vi "Outward.vi"(11 "64 in":refnum<class "Border.lvclass">) -> (1 "Direction":i32, 2 "Replicated out":refnum<class "Border.lvclass">, 3 "64 out":refnum<class "Border.lvclass">)   [LabVIEW 2015, in "Border.lvclass"]
uses:
  Border.lvclass
  Type Defs/Direction Enum.ctl
  Border.lvclass/Border.ctl
  SubVIs/Read-Only Globals.vi
  SubVIs/Globals (private).vi
  Square/Square.lvclass
  Type Defs/SB Type Defs.lvlib
  Common/Common.lvlib
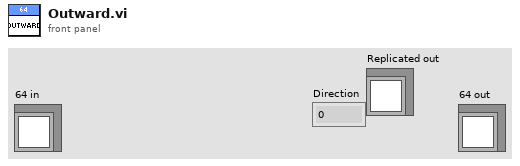
[diagram p1: front panel]
types:
  T1 = typedef "SB Type Defs.lvlib/Direction Enum.ctl" = enum16{"NW", "N", "NE", "E", "SE", "S", "SW", "W"}
  T2 = typedef "Common.lvlib/Position.ctl" = cluster{"Column":i32, "Row":i32}
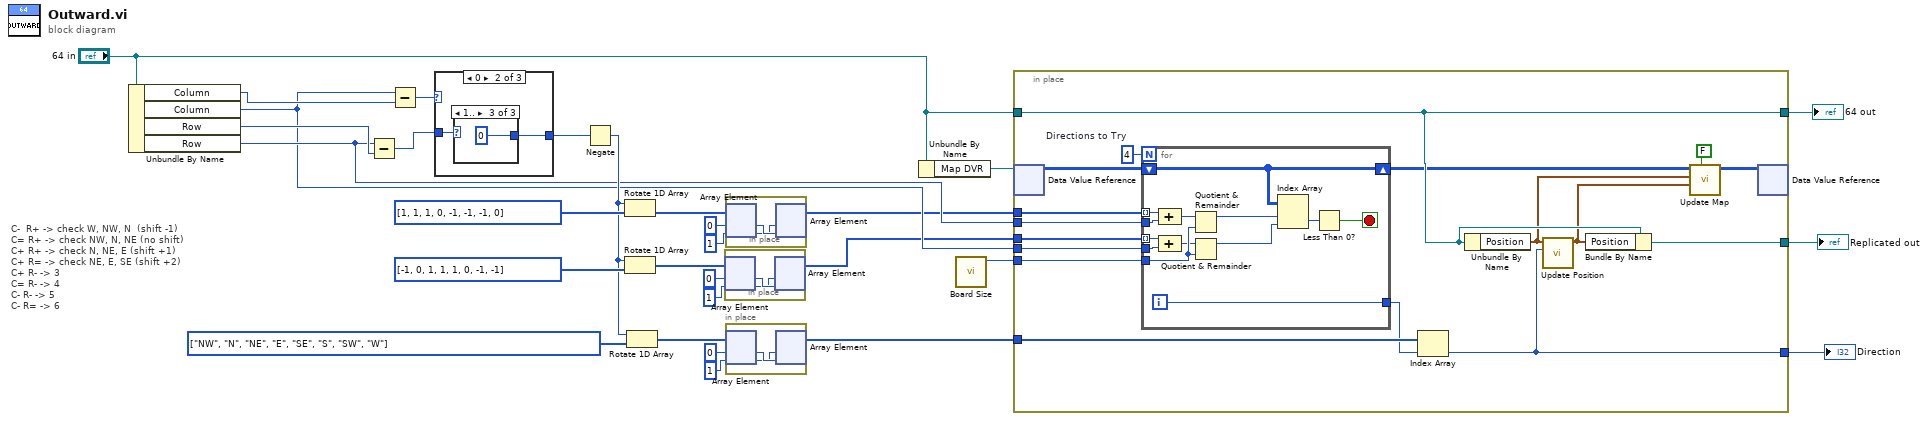
[diagram p0: block diagram]
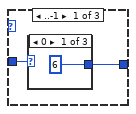
[diagram p2: hidden frame]
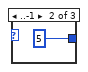
[diagram p3: hidden frame]
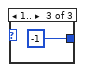
[diagram p4: hidden frame]
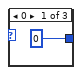
[diagram p5: hidden frame]
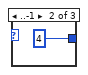
[diagram p6: hidden frame]
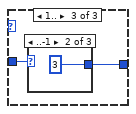
[diagram p7: hidden frame]
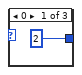
[diagram p8: hidden frame]
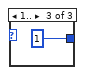
[diagram p9: hidden frame]
diagram:
  w22 = T1[] [enum."NW", enum."N", enum."NE", enum."E", enum."SE", enum."S", enum."SW", enum."W"] items=["NW", "N", "NE", "E", "SE", "S", "SW", "W"]
  # "C-  R+ -> check W, NW, N  (shift -1)\nC= R+ -> check NW, N, NE (no shift)\nC+ R+ -> check N, NE, E (shift +1)\nC+ R= -> check NE, E, SE (shift +2)\nC+ R- -> 3\nC= R- -> 4\nC- R- -> 5\nC- R= -> 6"
  n1 = Unbundle By Name("64 in") -> ("Column"=w29:i32, "Column"=w18:i32, "Row"=w23:i32, "Row"=w19:i32)
  n2 = Subtract(x=w19, y=w23) -> (x-y=w24:i32)
  n3 = Subtract(x=w18, y=w29) -> (x-y=w25:i32)
  n4 = case shown="0" w25 {
    tunnel: w24 -> [w31 w36 w41]
    tunnel: [w30 w35 w40] -> w13
    frame ..-1 {
      n5 = case shown="0" w31 {
        tunnel: [6 5 -1] -> w30
        frame 0 {
        }
        frame ..-1 {
        }
        frame 1.. {
        }
      }
    }
    frame 0 {
      n6 = case shown="1.." w36 {
        tunnel: [0 4 0] -> w35
        frame 0 {
        }
        frame ..-1 {
        }
        frame 1.. {
        }
      }
    }
    frame 1.. {
      n7 = case shown="..-1" w41 {
        tunnel: [2 3 1] -> w40
        frame 0 {
        }
        frame ..-1 {
        }
        frame 1.. {
        }
      }
    }
  }
  n8 = Negate(x=w13) -> (-x=w20:i32)
  n9 = Rotate 1D Array(1:i32[] [1, 1, 1, 0, -1, -1, -1, 0], 2:w20) -> (0:w10:i32[])
  n10 = Rotate 1D Array(1:i32[] [-1, 0, 1, 1, 1, 0, -1, -1], 2:w20) -> (0:w8:i32[])
  n11 = Rotate 1D Array(1:w22, 2:w20) -> (0:w12:T1[])
  n12 = in-place {
    n13 = in-place-array #1(w8, 0, 1) -> (w46:i32, w45:i32)
    n14 = in-place-array #1(w45, w46) -> (w7:i32[])  [unwired: 2 out]
  }
  n15 = in-place {
    n16 = in-place-array #2(w10, 0, 1) -> (w48:i32, w47:i32)
    n17 = in-place-array #2(w47, w48) -> (w9:i32[])  [unwired: 2 out]
  }
  n18 = in-place {
    n19 = in-place-array #3(w12, 0, 1) -> (w50:T1, w49:T1)
    n20 = in-place-array #3(w49, w50) -> (w11:T1[])  [unwired: 2 out]
  }
  n21 = Unbundle By Name("64 in") -> ("Map DVR"=w17:refnum<data-value>)
  n22 = call "Board Size.vi"() -> ("Board Size"=w28:i32)  [unwired: 11 in]
  n23 = in-place {
    in-place-border: w28 -> [w67]
    in-place-border: w9 -> [w66]
    in-place-border: w7 -> [w65]
    in-place-border: w11 -> [w63]
    in-place-border: [w57] -> w21
    in-place-border: w19 -> [w61]
    in-place-border: w18 -> [w60]
    in-place-border: "64 in" -> [w56]
    in-place-border: [w56] -> w15
    in-place-border: [w58] -> w14
    w64 = 4  # Directions to Try
    n24 = in-place-dvr #4(w17) -> (w59:i32[][])  [unwired: 1 out]
    n25 = for {
      N: w64 -> [_]
      tunnel: w66 -> [w80] mode=indexing
      tunnel: w65 -> [w79] mode=indexing
      tunnel: w67 -> [w78]
      tunnel: [w75] -> w62
      tunnel: w61 -> [w71]
      tunnel: w60 -> [w70]
      shift-right: [w68] -> w55
      shift-left: w59 -> [w68]
      i -> [w75]
      stop <- w72 stop-if-true
      n26 = Compound Arithmetic op=ADD(w80, w71) -> (w77:i32)
      n27 = Compound Arithmetic op=ADD(w79, w70) -> (w76:i32)
      n28 = Quotient & Remainder(x=w77, y=w78) -> (x-y*floor(x/y)=w74:i32)  [unwired: 1 out]
      n29 = Quotient & Remainder(x=w76, y=w78) -> (x-y*floor(x/y)=w73:i32)  [unwired: 1 out]
      n30 = Index Array(array=w68, index (row)=w74, index (col)=w73) -> (element=w69:i32)
      n31 = Less Than 0?(x=w69) -> (x < 0?=w72:bool)
    }
    n32 = Index Array(array=w63, index=w62) -> (element=w57:T1)
    n33 = Unbundle By Name(w56) -> ("Position"=w53:T2)
    n34 = call "Update Position.vi"("Direction"=w57, "Position in"=w53) -> ("Position out"=w52:T2)  [unwired: 9 in]
    n35 = Bundle By Name(cluster=w56, "Position"=w52) -> (w58:refnum<class "Border.lvclass">)
    n36 = call "Update Map.vi"("Moved?"=FALSE, "New Position"=w52, "Old Position"=w53, "Map in"=w55) -> ("Map"=w54:i32[][])  [unwired: 7 in]
    n37 = in-place-dvr #4(w54) -> ()  [unwired: 2 out]
  }
  "64 out" <- w15
  "Direction" <- w21
  "Replicated out" <- w14
